vi "Get BuildSpec Destinaton Path.vi"(8 "error in":errorcluster, 11 "Project Path":path) -> (0 "error out":errorcluster, 3 "Build path":path)   [LabVIEW 2026, in "NIVS_CDEW_MetaDataObj.lvclass"]
uses:
  NIVS_CDEW_MetaDataObj.lvclass
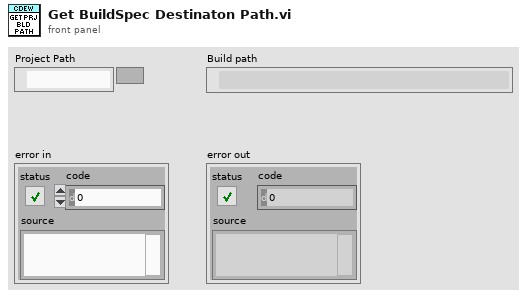
[diagram p1: front panel]
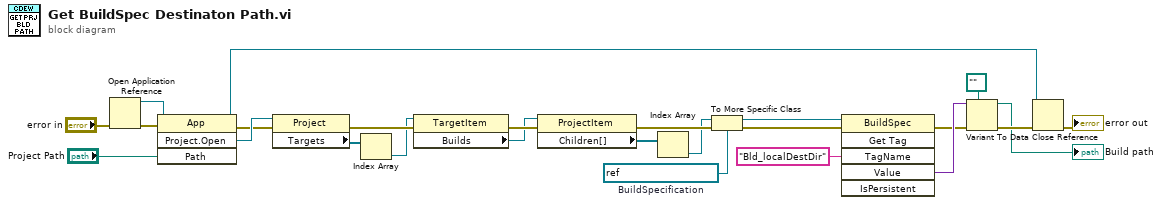
[diagram p0: block diagram]
diagram:
  w11 = refnum<vi> refnum  # BuildSpecification
  n1 = Open Application Reference(8:"error in") -> (0:w25:errorcluster, 3:w22:refnum<vi>)  [unwired: 3 in]
  n2 = invoke class="App" method="Project.Open"(reference=w22, error in=w25, "Path"="Project Path") -> (reference out=w17:refnum<vi>, error out=w20:errorcluster, "Project:Open"=w24:refnum<vi>)  [unwired: 1 in, 1 out]
  n3 = property class="Project"(reference=w24, error in=w20) -> (error out=w19:errorcluster, "Targets"=w15:refnum<vi>[])  [unwired: 1 out]
  n4 = Index Array(array=w15) -> (element=w14:refnum<vi>)  [unwired: 1 in]
  n5 = property class="TargetItem"(reference=w14, error in=w19) -> (error out=w13:errorcluster, "Builds"=w12:refnum<vi>)  [unwired: 1 out]
  n6 = property class="ProjectItem"(reference=w12, error in=w13) -> (error out=w10:errorcluster, "Children[]"=w9:refnum<vi>[])  [unwired: 1 out]
  n7 = Index Array(array=w9) -> (element=w8:refnum<vi>)  [unwired: 1 in]
  n8 = To More Specific Class(target class=w11, reference=w8, error in=w10) -> (specific class reference=w7:refnum<vi>, error out=w3:errorcluster)
  n9 = invoke class="BuildSpec" method="Get Tag"(reference=w7, error in=w3, "TagName"="Bld_localDestDir" ("Tag Name")) -> (error out=w2:errorcluster, "Value"=w5:variant)  [unwired: 3 in, 4 out]
  n10 = Variant To Data(error in=w2, type=path "", Variant=w5) -> (data=→"Build path":path, error out=w18:errorcluster)
  n11 = Close Reference(reference=w17, error in (no error)=w18) -> (error out=→"error out":errorcluster)
